vi "MultiStationGasMeter_Rev3.vi"() -> ()   [LabVIEW 2014]
uses:
  <vilib>/DAQmx/read.llb/DAQmx Read (Analog 1D DBL NChan 1Samp).vi
  <vilib>/DAQmx/miscellaneous.llb/DAQmx Fill In Error Info.vi
panel:
  in  "Rate Threshold (V)":dbl=0.02
  in  "HeatingValueLP 3":dbl=990.0 min=900.0 max=2600.0 step=1.0
  in  "HeatingValueNG 3":dbl=990.0 min=900.0 max=1200.0 step=1.0
  in  "Start ANSI 3":bool
  out "ANSI Average (BTU/hr) 3":dbl format="%#_5g"
  out "30 Second Average (BTU/hr) 3":dbl format="%#_5g"
  out "15 Second Average (BTU/hr) 3":dbl format="%#_5g"
  out "Signal 3":bool
  out "CF/HR 3":dbl format="%#_2g"
  out "HV 3":dbl
  out "Meter ID 3":dbl
  out "Gas 3":string
  out "DisplayChart 3":cluster{"Flow Rate":dbl}(graph)
  out "Flow Rate 3":dbl format="%#_5g"
  in  "HeatingValueLP 2":dbl=990.0 min=900.0 max=2600.0 step=1.0
  in  "Start ANSI 2":bool
  out "ANSI Average (BTU/hr) 2":dbl format="%#_5g"
  out "30 Second Average (BTU/hr) 2":dbl format="%#_5g"
  out "15 Second Average (BTU/hr) 2":dbl format="%#_5g"
  out "Signal 2":bool
  out "CF/HR 2":dbl format="%#_2g"
  out "HV 2":dbl
  in  "HeatingValueNG 2":dbl=990.0 min=900.0 max=1200.0 step=1.0
  out "Meter ID 2":dbl
  out "Gas 2":string
  out "DisplayChart 2":cluster{"Flow Rate":dbl}(graph)
  out "Flow Rate 2":dbl format="%#_5g"
  out "ANSI Placeholder 3":dbl
  out "Start Time ANSI 3":dbl
  out "ANSI Placeholder 2":dbl
  out "Start Time ANSI 2":dbl
  out "Meter 6 Present":bool
  out "Meter 5 Present":bool
  out "Meter 4 Present":bool
  out "Meter 3 Present":bool
  out "Meter 2 Present":bool
  out "Meter 1 Present":bool
  out "Meter Type 6":string
  out "Meter Type 2":string
  out "Meter Type 4":string
  out "Meter Type 5":string
  out "Meter Type 3":string
  out "Meter Type 1":string
  out "Meter 6 Size":dbl
  out "Meter 5 Size":dbl
  out "Meter 4 Size":dbl
  out "Meter 3 Size":dbl
  out "Meter 2 Size":dbl
  out "Meter 1 Size":dbl
  out "ANSI Placeholder":dbl
  out "Start Time ANSI":dbl
  in  "Start ANSI":bool
  out "ANSI Average (BTU/hr)":dbl format="%#_5g"
  out "30 Second Average (BTU/hr)":dbl format="%#_5g"
  out "15 Second Average (BTU/hr)":dbl format="%#_5g"
  out "Reference6":dbl
  out "Reference5":dbl
  out "Reference4":dbl
  out "Reference3":dbl
  out "Reference2":dbl
  out "Reference1":dbl
  out "Time":dbl
  out "Num Record":dbl
  in  "HeatingValueLP":dbl=2450.0 min=2400.0 max=2600.0 step=1.0
  out "Output 6":dbl min=0.0 max=5.0 step=0.01
  out "Output 5":dbl min=0.0 max=5.0 step=0.01
  out "Output 4":dbl min=0.0 max=5.0 step=0.01
  out "Output 3":dbl min=0.0 max=5.0 step=0.01
  out "Output 2":dbl min=0.0 max=5.0 step=0.01
  out "Output 1":dbl min=0.0 max=5.0 step=0.01
  out "Signal":bool
  in  "Record":bool
  out "File Path":path
  out "CF/HR":dbl format="%#_2g"
  out "HV":dbl
  in  "HeatingValueNG":dbl=990.0 min=900.0 max=1200.0 step=1.0
  out "Meter ID":dbl
  out "Gas":string
  out "DisplayChart":cluster{"Flow Rate":dbl}(graph)
  out "Flow Rate":dbl format="%#_5g"
  # "STATION 1"
  # "STATION 2"
  # "STATION 3"
  # "Heating Value"
  # "Heating Value"
  # "Heating Value"
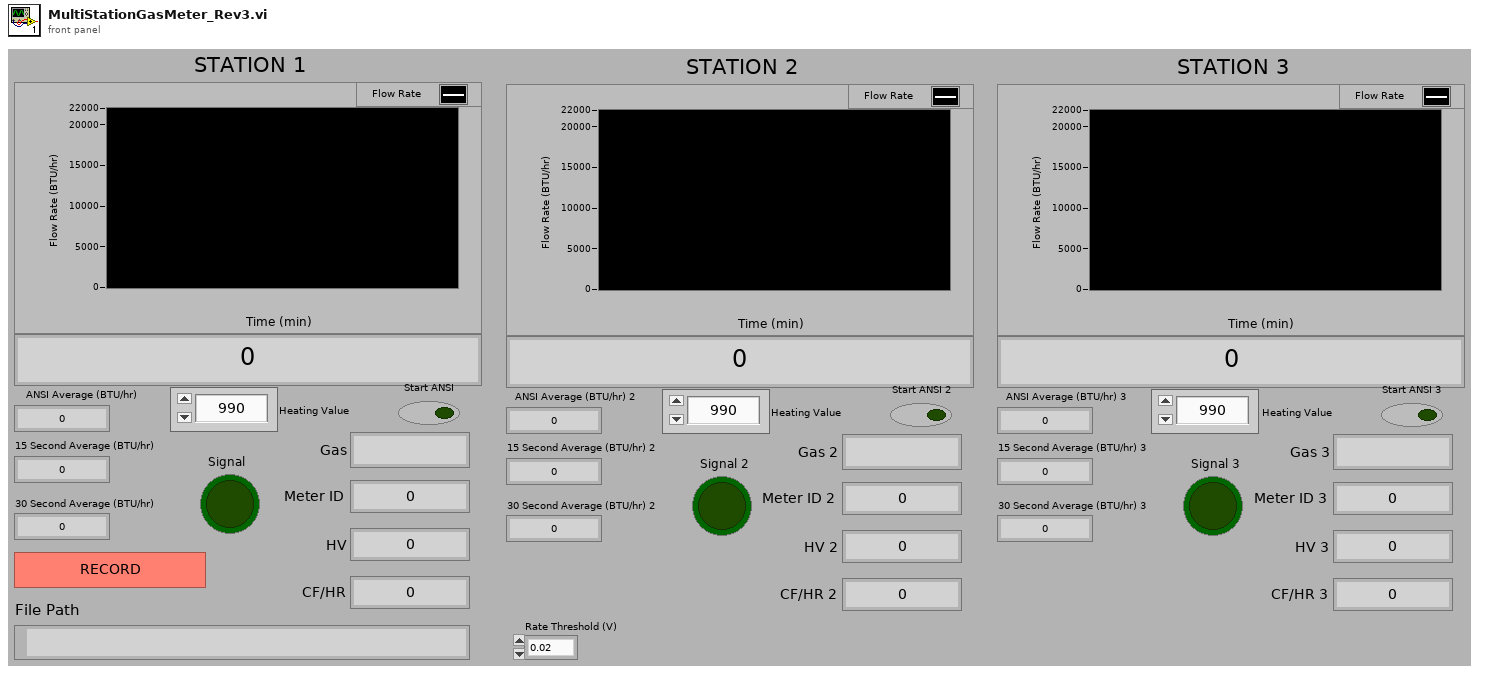
[diagram p1: front panel]
types:
  T1 = enum16{"open", "replace", "create", "open or create", "replace or create", "replace or create with confirmation"}
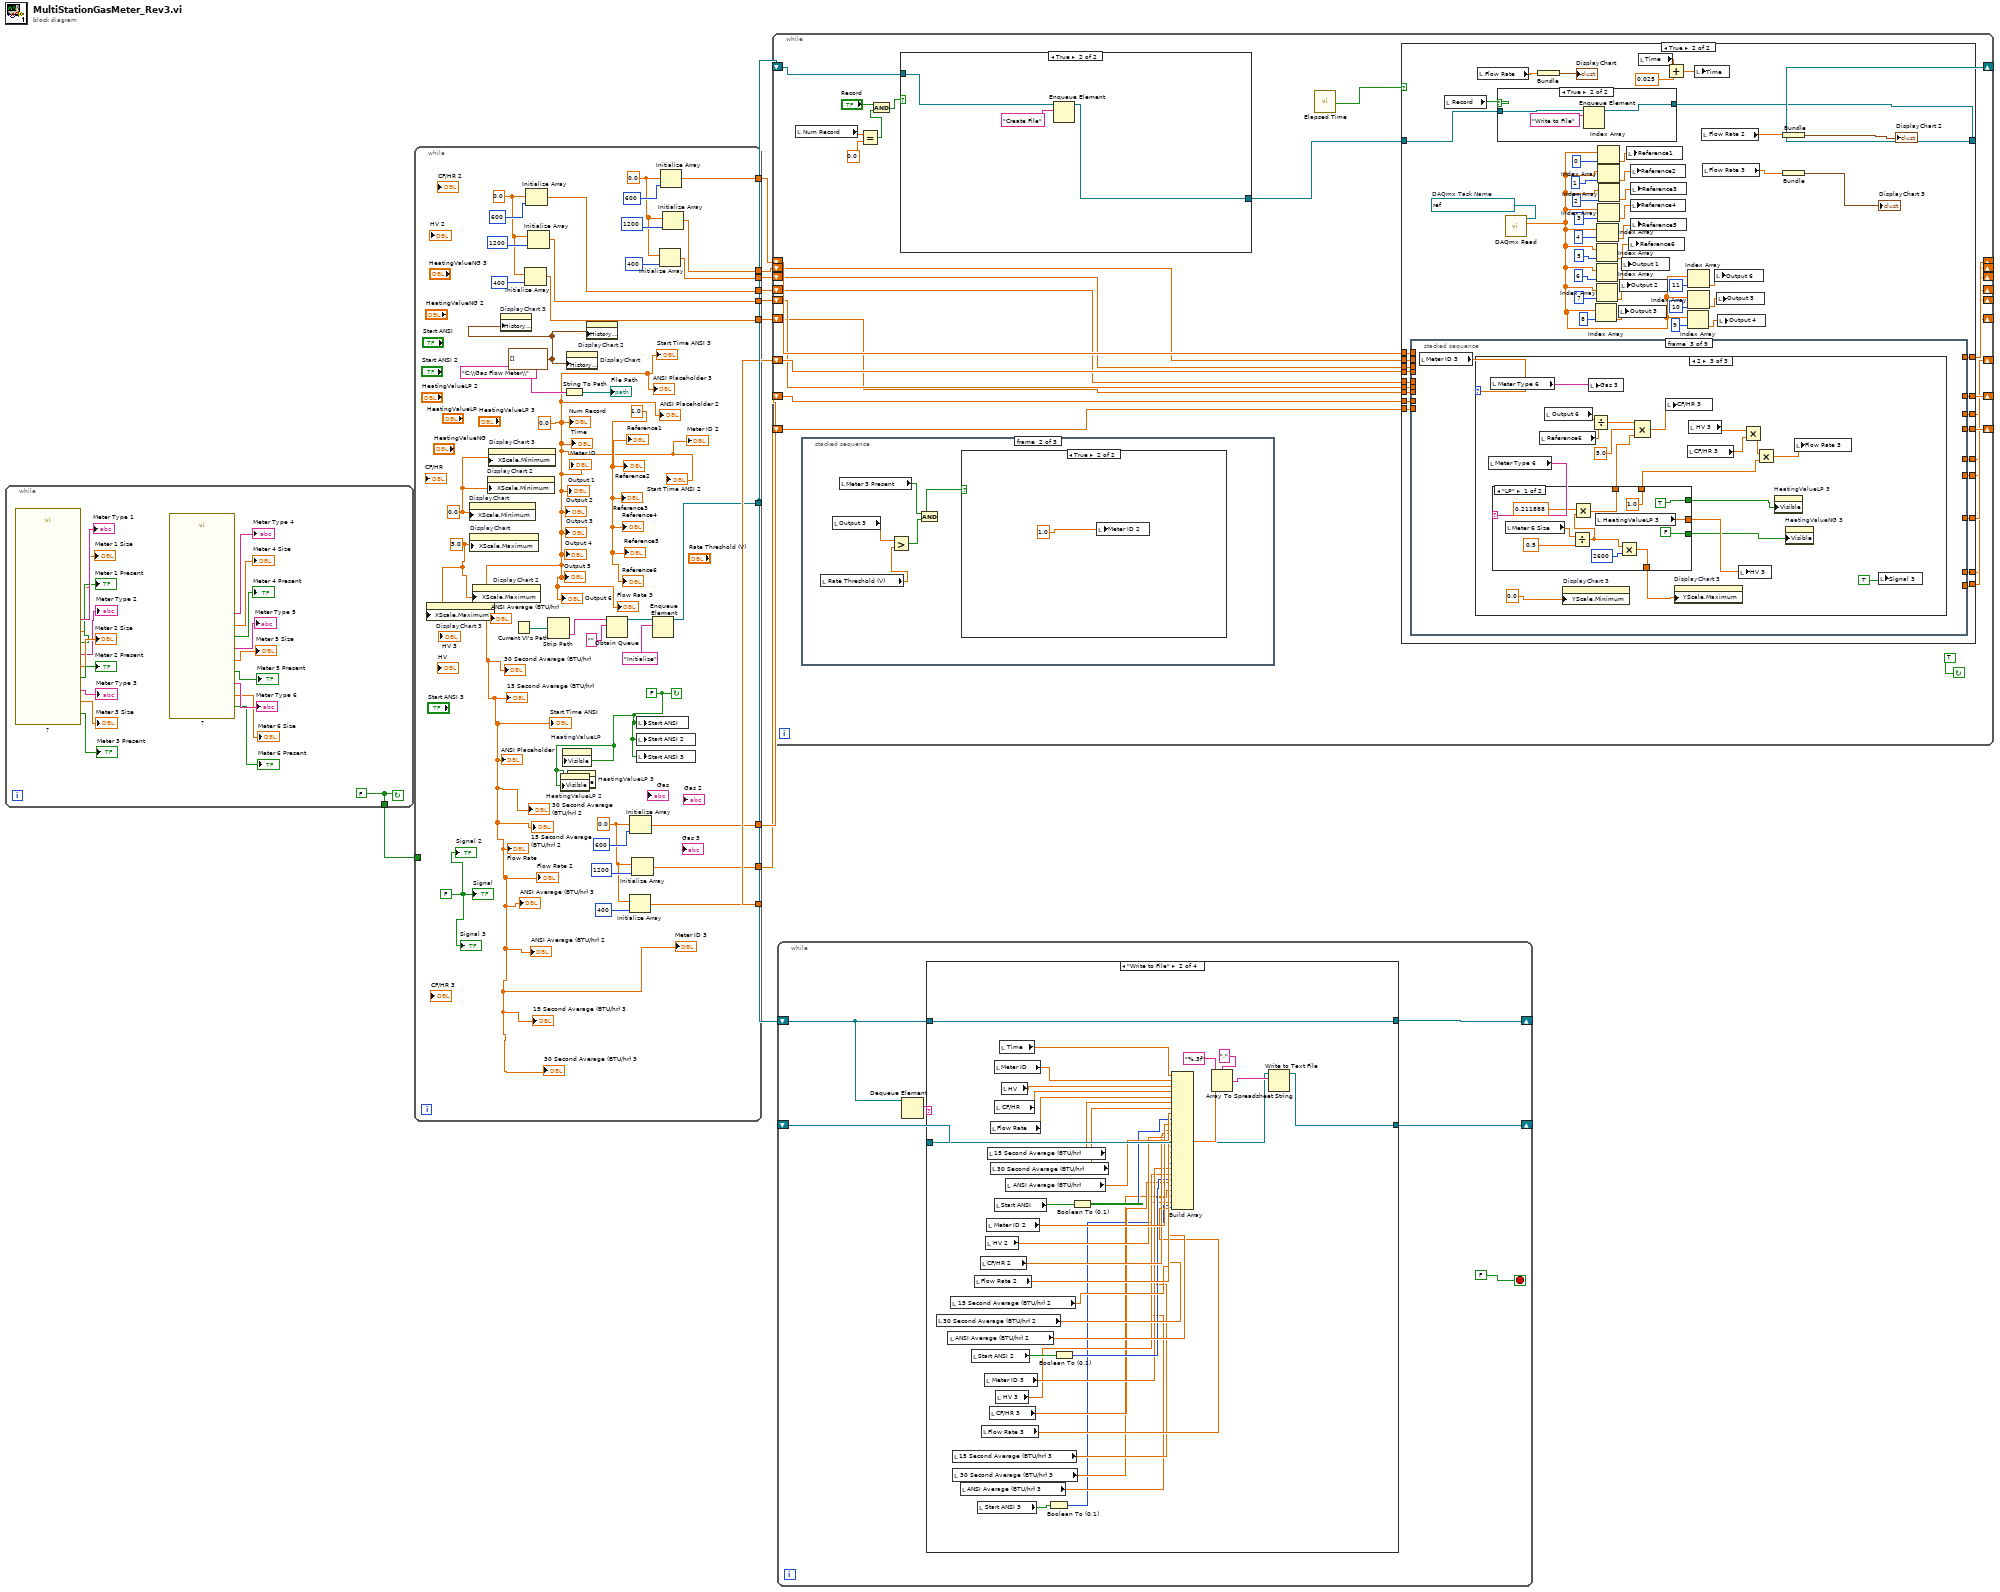
[diagram p0: block diagram]
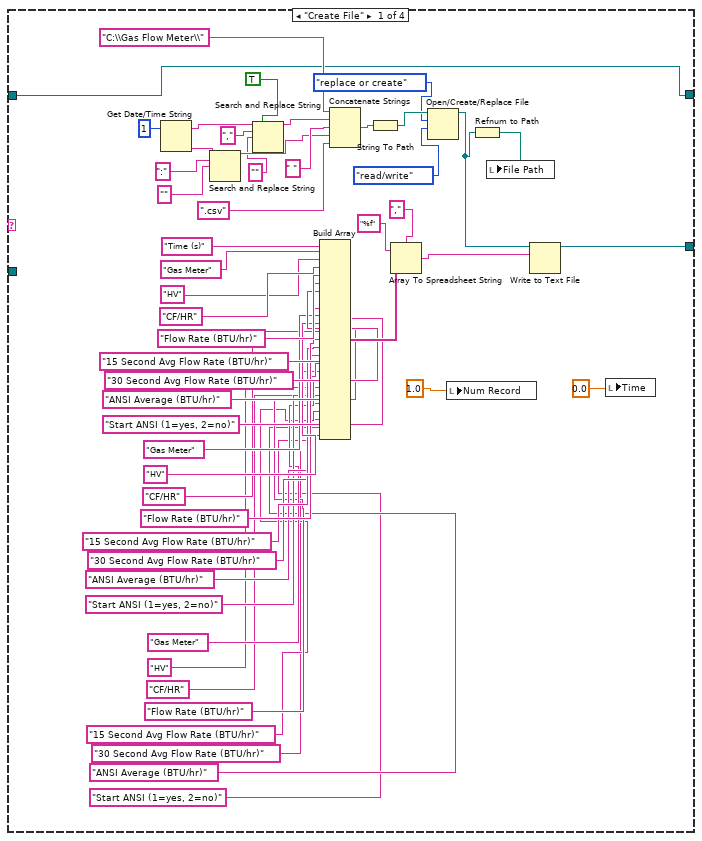
[diagram p2: hidden frame]
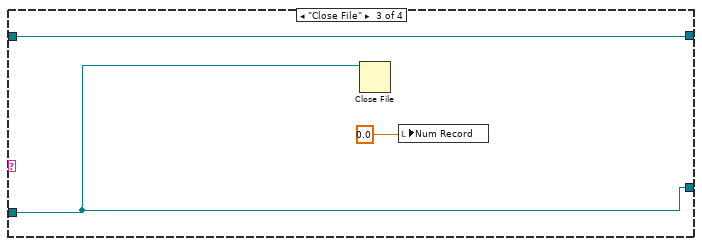
[diagram p3: hidden frame]
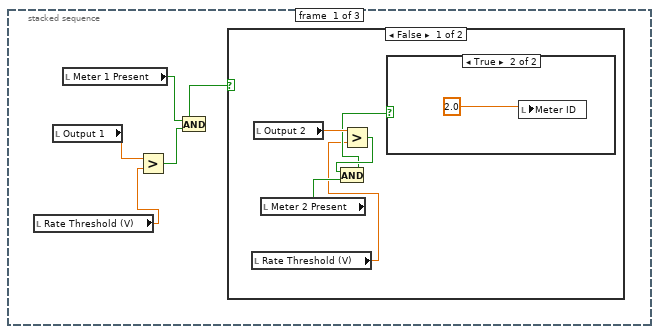
[diagram p5: hidden frame]
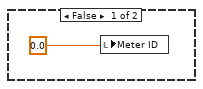
[diagram p6: hidden frame]
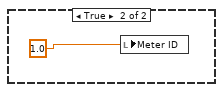
[diagram p7: hidden frame]
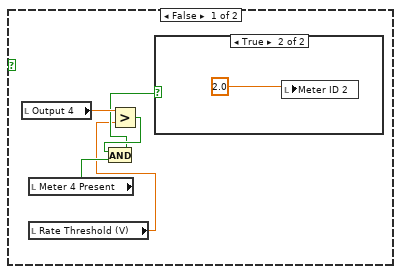
[diagram p8: hidden frame]
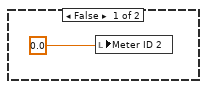
[diagram p9: hidden frame]
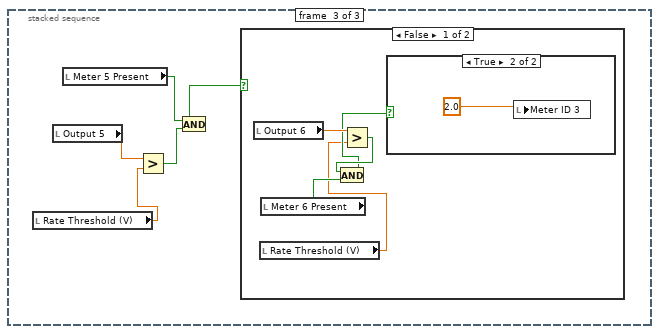
[diagram p10: hidden frame]
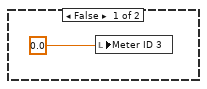
[diagram p11: hidden frame]
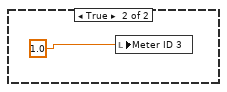
[diagram p12: hidden frame]
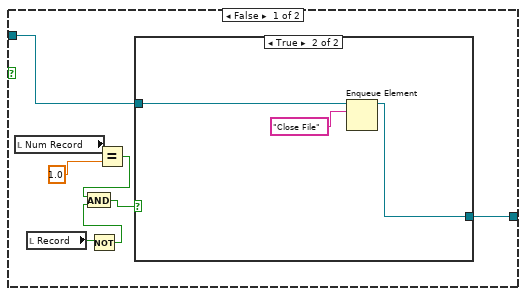
[diagram p13: hidden frame]
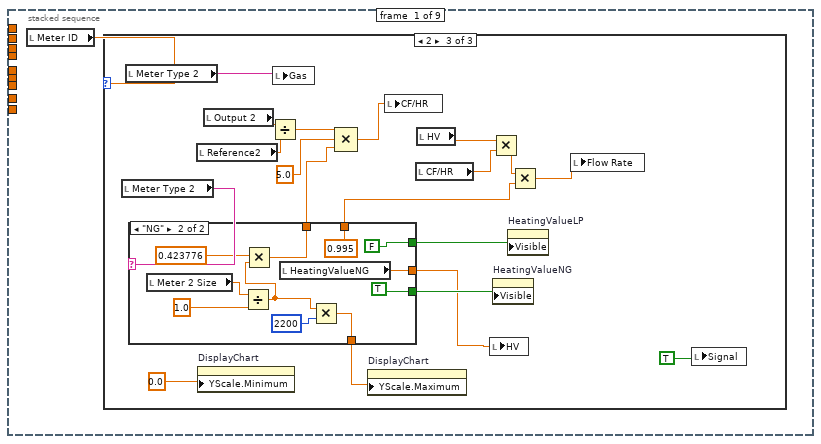
[diagram p16: hidden frame]
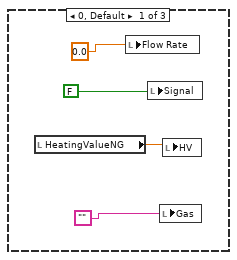
[diagram p17: hidden frame]
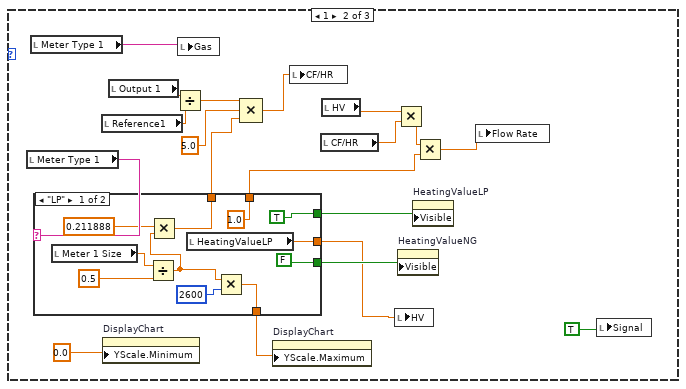
[diagram p18: hidden frame]
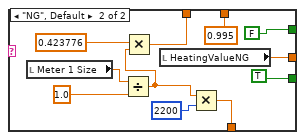
[diagram p19: hidden frame]
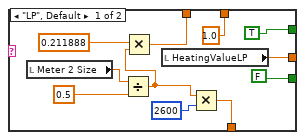
[diagram p20: hidden frame]
diagram:
  n1 = while {
    tunnel: [w29] -> w7
    stop <- w29 continue-if-true
    w29 = FALSE
    n2 = call "?"() -> ("Meter 3 Present?"=→"Meter 3 Present":bool, "Meter Size 3 (SLPM)"=→"Meter 3 Size":dbl, "Meter Type 3 (LP/NG)"=→"Meter Type 3":string, "Meter 2 Present?"=→"Meter 2 Present":bool, "Meter Size 2 (SLPM)"=→"Meter 2 Size":dbl, "Meter Type 2 (LP/NG)"=→"Meter Type 2":string, "Meter 1 Present?"=→"Meter 1 Present":bool, "Meter Size 1 (SLPM)"=→"Meter 1 Size":dbl, "Meter Type 1 (LP/NG)"=→"Meter Type 1":string)  [unwired: 9 in, 2 out]
    n3 = call "?"() -> ("Meter 6 Present?"=→"Meter 6 Present":bool, "Meter Size 6 (SLPM)"=→"Meter 6 Size":dbl, "Meter Type 6 (LP/NG)"=→"Meter Type 6":string, "Meter 5 Present?"=→"Meter 5 Present":bool, "Meter Size 5 (SLPM)"=→"Meter 5 Size":dbl, "Meter Type 5 (LP/NG)"=→"Meter Type 5":string, "Meter 4 Present?"=→"Meter 4 Present":bool, "Meter Size 4 (SLPM)"=→"Meter 4 Size":dbl, "Meter Type 4 (LP/NG)"=→"Meter Type 4":string)  [unwired: 9 in, 2 out]
  }
  n4 = while {
    tunnel: [w60] -> w11
    tunnel: [w56] -> w10
    tunnel: [w55] -> w9
    tunnel: [w52] -> w8
    tunnel: w7 -> [_]
    tunnel: [w47] -> w6
    tunnel: [w46] -> w5
    tunnel: [w45] -> w4
    tunnel: [w40] -> w3
    tunnel: [w39] -> w2
    tunnel: [w38] -> w1
    stop <- w36 continue-if-true
    w42 = 0.0
    w49 = 0.0
    w35 = FALSE
    w54 = 0.0
    w31 = 5.0
    w32 = 0.0
    w59 = 1.0
    w34 = 0.0
    w33 = cluster{"[0]":dbl}[] []
    w36 = FALSE
    n5 = property on="DisplayChart 3" class="WFChart (strict)"("XScale.Maximum"=w31) -> ()  [unwired: 2 in, 2 out]
    n6 = property on="DisplayChart" class="WFChart (strict)"("XScale.Minimum"=w32) -> ()  [unwired: 2 in, 2 out]
    n7 = property on="DisplayChart" class="WFChart (strict)"("XScale.Maximum"=w31) -> ()  [unwired: 2 in, 2 out]
    n8 = property on="DisplayChart 2" class="WFChart (strict)"("XScale.Maximum"=w31) -> ()  [unwired: 2 in, 2 out]
    n9 = property on="DisplayChart 2" class="WFChart (strict)"("XScale.Minimum"=w32) -> ()  [unwired: 2 in, 2 out]
    n10 = property on="DisplayChart 3" class="WFChart (strict)"("XScale.Minimum"=w32) -> ()  [unwired: 2 in, 2 out]
    n11 = property on="DisplayChart 3" class="WFChart (strict)"("History Data"=w33) -> ()  [unwired: 2 in, 2 out]
    n12 = Current VI's Path() -> (path=w65:path)
    n13 = Initialize Array(w42, 400) -> (w38:dbl[])
    n14 = Initialize Array(w42, 600) -> (w40:dbl[])
    n15 = Initialize Array(w42, 1200) -> (w39:dbl[])
    n16 = Strip Path(path=w65) -> (name=w63:string)  [unwired: 1 out]
    n17 = property on="HeatingValueLP 2" class="DigNum (strict)"("Visible"=w36) -> ()  [unwired: 2 in, 2 out]
    n18 = property on="HeatingValueLP" class="DigNum (strict)"("Visible"=w36) -> ()  [unwired: 2 in, 2 out]
    n19 = String To Path(string="C:\\Gas Flow Meter\\") -> (path=→"File Path":path)
    n20 = property on="DisplayChart" class="WFChart (strict)"("History Data"=w33) -> ()  [unwired: 2 in, 2 out]
    n21 = property on="HeatingValueLP 3" class="DigNum (strict)"("Visible"=w36) -> ()  [unwired: 2 in, 2 out]
    n22 = property on="DisplayChart 2" class="WFChart (strict)"("History Data"=w33) -> ()  [unwired: 2 in, 2 out]
    n23 = Obtain Queue(name (unnamed)=w63, element data type="") -> (queue out=w61:refnum<queue>)  [unwired: 3 in, 2 out]
    n24 = Initialize Array(w54, 400) -> (w52:dbl[])
    n25 = Initialize Array(w54, 600) -> (w56:dbl[])
    n26 = Initialize Array(w54, 1200) -> (w55:dbl[])
    n27 = local write "Start ANSI"(w36) -> ()
    n28 = local write "Start ANSI 2"(w36) -> ()
    n29 = local write "Start ANSI 3"(w36) -> ()
    n30 = Enqueue Element(queue=w61, element="Initialize") -> (queue out=w60:refnum<queue>)  [unwired: 2 in, 2 out]
    n31 = Initialize Array(w49, 400) -> (w45:dbl[])
    n32 = Initialize Array(w49, 600) -> (w47:dbl[])
    n33 = Initialize Array(w49, 1200) -> (w46:dbl[])
    "Num Record" <- w34
    "Time" <- w34
    "Meter ID" <- w34
    "Output 1" <- w34
    "Output 2" <- w34
    "Output 3" <- w34
    "Output 4" <- w34
    "Output 5" <- w34
    "Output 6" <- w34
    "Reference1" <- w59
    "Reference2" <- w59
    "Reference3" <- w59
    "Reference4" <- w59
    "Reference5" <- w59
    "Reference6" <- w59
    "30 Second Average (BTU/hr)" <- w34
    "15 Second Average (BTU/hr)" <- w34
    "ANSI Average (BTU/hr)" <- w34
    "Start Time ANSI" <- w34
    "ANSI Placeholder" <- w34
    "Flow Rate" <- w34
    "Signal" <- w35
    "Start Time ANSI 3" <- w34
    "ANSI Placeholder 3" <- w34
    "ANSI Placeholder 2" <- w34
    "Start Time ANSI 2" <- w34
    "Signal 2" <- w35
    "Flow Rate 2" <- w34
    "ANSI Average (BTU/hr) 2" <- w34
    "Meter ID 2" <- w34
    "30 Second Average (BTU/hr) 2" <- w34
    "15 Second Average (BTU/hr) 2" <- w34
    "Signal 3" <- w35
    "Flow Rate 3" <- w34
    "Meter ID 3" <- w34
    "ANSI Average (BTU/hr) 3" <- w34
    "15 Second Average (BTU/hr) 3" <- w34
    "30 Second Average (BTU/hr) 3" <- w34
  }
  n34 = while {
    shift-right: [w92] -> _
    shift-left: w11 -> [w85]
    shift-right: [w91] -> _
    shift-left: w10 -> [w89]
    shift-right: [w90] -> _
    shift-left: w9 -> [w88]
    shift-right: [w87] -> _
    shift-left: w8 -> [w86]
    shift-right: [w77] -> _
    shift-left: w6 -> [w78]
    shift-right: [w75] -> _
    shift-left: w5 -> [w76]
    shift-right: [w73] -> _
    shift-left: w4 -> [w74]
    shift-right: [w71] -> _
    shift-left: w3 -> [w72]
    shift-right: [w69] -> _
    shift-left: w2 -> [w70]
    shift-right: [w67] -> _
    shift-left: w1 -> [w68]
    stop <- TRUE continue-if-true
    n35 = local read "Num Record"() -> (w81:dbl)
    n36 = stacked-sequence {
      frame #0 {
        n37 = local read "Rate Threshold (V)"() -> (w95:dbl)
        n38 = local read "Output 1"() -> (w99:dbl)
        n39 = local read "Meter 1 Present"() -> (w97:bool)
        n40 = Greater?(x=w99, y=w95) -> (0:w98:bool)
        n41 = And(x=w97, y=w98) -> (x .and. y?=w96:bool)
        n42 = case shown="False" w96 {
          frame False {
            n43 = local read "Rate Threshold (V)"() -> (w100:dbl)
            n44 = local read "Output 2"() -> (w104:dbl)
            n45 = local read "Meter 2 Present"() -> (w103:bool)
            n46 = Greater?(x=w104, y=w100) -> (0:w102:bool)
            n47 = And(x=w102, y=w103) -> (x .and. y?=w101:bool)
            n48 = case shown="True" w101 {
              frame False {
                n49 = local write "Meter ID"(0.0) -> ()
              }
              frame True {
                n50 = local write "Meter ID"(2.0) -> ()
              }
            }
          }
          frame True {
            n51 = local write "Meter ID"(1.0) -> ()
          }
        }
      }
      frame #1 {
        n52 = local read "Rate Threshold (V)"() -> (w108:dbl)
        n53 = local read "Output 3"() -> (w112:dbl)
        n54 = local read "Meter 3 Present"() -> (w110:bool)
        n55 = Greater?(x=w112, y=w108) -> (0:w111:bool)
        n56 = And(x=w110, y=w111) -> (x .and. y?=w109:bool)
        n57 = case shown="True" w109 {
          frame False {
            n58 = local read "Output 4"() -> (w117:dbl)
            n59 = local read "Meter 4 Present"() -> (w116:bool)
            n60 = local read "Rate Threshold (V)"() -> (w113:dbl)
            n61 = Greater?(x=w117, y=w113) -> (0:w115:bool)
            n62 = And(x=w115, y=w116) -> (x .and. y?=w114:bool)
            n63 = case shown="True" w114 {
              frame False {
                n64 = local write "Meter ID 2"(0.0) -> ()
              }
              frame True {
                n65 = local write "Meter ID 2"(2.0) -> ()
              }
            }
          }
          frame True {
            n66 = local write "Meter ID 2"(1.0) -> ()
          }
        }
      }
      frame #2 {
        n67 = local read "Rate Threshold (V)"() -> (w121:dbl)
        n68 = local read "Output 5"() -> (w125:dbl)
        n69 = local read "Meter 5 Present"() -> (w123:bool)
        n70 = Greater?(x=w125, y=w121) -> (0:w124:bool)
        n71 = And(x=w123, y=w124) -> (x .and. y?=w122:bool)
        n72 = case shown="False" w122 {
          frame False {
            n73 = local read "Output 6"() -> (w130:dbl)
            n74 = local read "Rate Threshold (V)"() -> (w126:dbl)
            n75 = local read "Meter 6 Present"() -> (w129:bool)
            n76 = Greater?(x=w130, y=w126) -> (0:w128:bool)
            n77 = And(x=w128, y=w129) -> (x .and. y?=w127:bool)
            n78 = case shown="True" w127 {
              frame False {
                n79 = local write "Meter ID 3"(0.0) -> ()
              }
              frame True {
                n80 = local write "Meter ID 3"(2.0) -> ()
              }
            }
          }
          frame True {
            n81 = local write "Meter ID 3"(1.0) -> ()
          }
        }
      }
    }
    n82 = Equal?(x=w81, y=0.0) -> (x = y?=w80:bool)
    n83 = And(x="Record", y=w80) -> (x .and. y?=w79:bool)
    n84 = case shown="True" w79 {
      tunnel: w85 -> [w139 w147]
      tunnel: [w138 w146] -> w84
      frame False {
        n85 = local read "Num Record"() -> (w141:dbl)
        n86 = local read "Record"() -> (w135:bool)
        n87 = Not(x=w135) -> (.not. x?=w134:bool)
        n88 = Equal?(x=w141, y=1.0) -> (x = y?=w137:bool)
        n89 = And(x=w137, y=w134) -> (x .and. y?=w136:bool)
        n90 = case shown="True" w136 {
          tunnel: w139 -> [w142 w144]
          tunnel: [w142 w143] -> w138
          frame False {
          }
          frame True {
            n91 = Enqueue Element(queue=w144, element="Close File") -> (queue out=w143:refnum<queue>)  [unwired: 2 in, 2 out]
          }
        }
      }
      frame True {
        n92 = Enqueue Element(queue=w147, element="Create File") -> (queue out=w146:refnum<queue>)  [unwired: 2 in, 2 out]
      }
    }
    n93 = call "Elapsed Time"() -> ("Time has Elapsed"=w93:bool)  [unwired: 12 in, 7 out]
    n94 = case shown="True" w93 {
      tunnel: w84 -> [w158 w208]
      tunnel: [w158 w207] -> w92
      tunnel: w89 -> [w157 w180]
      tunnel: w88 -> [w156 w179]
      tunnel: [w157 w178] -> w91
      tunnel: [w156 w177] -> w90
      tunnel: w86 -> [w155 w176]
      tunnel: [w155 w175] -> w87
      tunnel: w78 -> [w152 w174]
      tunnel: [w152 w173] -> w77
      tunnel: w76 -> [w153 w172]
      tunnel: [w153 w171] -> w75
      tunnel: w74 -> [w154 w170]
      tunnel: [w154 w169] -> w73
      tunnel: w72 -> [w151 w168]
      tunnel: [w151 w167] -> w71
      tunnel: w70 -> [w150 w166]
      tunnel: [w150 w165] -> w69
      tunnel: w68 -> [w149 w164]
      tunnel: [w149 w163] -> w67
      frame False {
      }
      frame True {
        w206 = refnum<k21> "ReadFlowMeterIn"  # DAQmx Task Name
        n95 = stacked-sequence {
          tunnel: w180 -> [_ _ _ w500 _ _ _ _ _]
          tunnel: w179 -> [_ _ _ w499 _ _ _ _ _]
          tunnel: [_ _ _ w494 _ _ _ _ _] -> w178
          tunnel: [_ _ _ w490 _ _ _ _ _] -> w177
          tunnel: w176 -> [_ _ _ w484 _ _ _ _ _]
          tunnel: [_ _ _ w481 _ _ _ _ _] -> w175
          tunnel: w174 -> [_ _ _ _ w523 _ _ _ _]
          tunnel: [_ _ _ _ w510 _ _ _ _] -> w173
          tunnel: w172 -> [_ _ _ _ w517 _ _ _ _]
          tunnel: [_ _ _ _ w509 _ _ _ _] -> w171
          tunnel: w170 -> [_ _ _ _ w515 _ _ _ _]
          tunnel: [_ _ _ _ w508 _ _ _ _] -> w169
          tunnel: w168 -> [_ _ _ _ _ w544 _ _ _]
          tunnel: [_ _ _ _ _ w542 _ _ _] -> w167
          tunnel: w166 -> [_ _ _ _ _ w541 _ _ _]
          tunnel: [_ _ _ _ _ w539 _ _ _] -> w165
          tunnel: w164 -> [_ _ _ _ _ w538 _ _ _]
          tunnel: [_ _ _ _ _ w536 _ _ _] -> w163
          frame #0 {
            n96 = local read "Meter ID"() -> (w215:dbl)
            n97 = case shown="2" w215 {
              frame 0, Default {
                n98 = local read "HeatingValueNG"() -> (w219:dbl)
                n99 = local write "Flow Rate"(0.0) -> ()
                n100 = local write "Signal"(FALSE) -> ()
                n101 = local write "Gas"("") -> ()
                n102 = local write "HV"(w219) -> ()
              }
              frame 1 {
                n103 = local read "Meter Type 1"() -> (w228:string)
                n104 = local read "Meter Type 1"() -> (w222:string)
                n105 = case shown="\"LP\"" w228 {
                  tunnel: [w246 w257] -> w227
                  tunnel: [TRUE FALSE] -> w226
                  tunnel: [FALSE TRUE] -> w225
                  tunnel: [1.0 0.995] -> w224
                  tunnel: [w240 w251] -> w223
                  tunnel: [w239 w250] -> w221
                  frame "LP" {
                    n106 = local read "Meter 1 Size"() -> (w248:dbl)
                    n107 = Divide(x=w248, y=0.5) -> (x/y=w241:dbl)
                    n108 = Multiply(x=0.211888, y=w241) -> (x*y=w246:dbl)
                    n109 = local read "HeatingValueLP"() -> (w239:dbl)
                    n110 = Multiply(x=w241, y=2600) -> (x*y=w240:dbl)
                  }
                  frame "NG", Default {
                    n111 = local read "Meter 1 Size"() -> (w259:dbl)
                    n112 = Divide(x=w259, y=1.0) -> (x/y=w252:dbl)
                    n113 = Multiply(x=0.423776, y=w252) -> (x*y=w257:dbl)
                    n114 = local read "HeatingValueNG"() -> (w250:dbl)
                    n115 = Multiply(x=w252, y=2200) -> (x*y=w251:dbl)
                  }
                }
                n116 = local read "Reference1"() -> (w232:dbl)
                n117 = property on="DisplayChart" class="WFChart (strict)"("YScale.Minimum"=0.0) -> ()  [unwired: 2 in, 2 out]
                n118 = local read "Output 1"() -> (w233:dbl)
                n119 = Divide(x=w233, y=w232) -> (x/y=w230:dbl)
                n120 = local write "Gas"(w222) -> ()
                n121 = Compound Arithmetic op=MULTIPLY(w230, 5.0, w227) -> (w220:dbl)
                n122 = property on="DisplayChart" class="WFChart (strict)"("YScale.Maximum"=w223) -> ()  [unwired: 2 in, 2 out]
                n123 = local write "CF/HR"(w220) -> ()
                n124 = local read "CF/HR"() -> (w235:dbl)
                n125 = local read "HV"() -> (w234:dbl)
                n126 = local write "HV"(w221) -> ()
                n127 = Multiply(x=w234, y=w235) -> (x*y=w236:dbl)
                n128 = property on="HeatingValueNG" class="DigNum (strict)"("Visible"=w225) -> ()  [unwired: 2 in, 2 out]
                n129 = property on="HeatingValueLP" class="DigNum (strict)"("Visible"=w226) -> ()  [unwired: 2 in, 2 out]
                n130 = Multiply(x=w236, y=w224) -> (x*y=w237:dbl)
                n131 = local write "Flow Rate"(w237) -> ()
                n132 = local write "Signal"(TRUE) -> ()
              }
              frame 2 {
                n133 = local read "Meter Type 2"() -> (w269:string)
                n134 = local read "Meter Type 2"() -> (w263:string)
                n135 = case shown="\"NG\"" w269 {
                  tunnel: [w287 w298] -> w268
                  tunnel: [TRUE FALSE] -> w267
                  tunnel: [FALSE TRUE] -> w266
                  tunnel: [1.0 0.995] -> w265
                  tunnel: [w281 w292] -> w264
                  tunnel: [w280 w291] -> w262
                  frame "LP", Default {
                    n136 = local read "Meter 2 Size"() -> (w289:dbl)
                    n137 = Divide(x=w289, y=0.5) -> (x/y=w282:dbl)
                    n138 = Multiply(x=0.211888, y=w282) -> (x*y=w287:dbl)
                    n139 = local read "HeatingValueLP"() -> (w280:dbl)
                    n140 = Multiply(x=w282, y=2600) -> (x*y=w281:dbl)
                  }
                  frame "NG" {
                    n141 = local read "Meter 2 Size"() -> (w300:dbl)
                    n142 = Divide(x=w300, y=1.0) -> (x/y=w293:dbl)
                    n143 = Multiply(x=0.423776, y=w293) -> (x*y=w298:dbl)
                    n144 = local read "HeatingValueNG"() -> (w291:dbl)
                    n145 = Multiply(x=w293, y=2200) -> (x*y=w292:dbl)
                  }
                }
                n146 = local read "Reference2"() -> (w273:dbl)
                n147 = property on="DisplayChart" class="WFChart (strict)"("YScale.Minimum"=0.0) -> ()  [unwired: 2 in, 2 out]
                n148 = local read "Output 2"() -> (w274:dbl)
                n149 = Divide(x=w274, y=w273) -> (x/y=w271:dbl)
                n150 = local write "Gas"(w263) -> ()
                n151 = Compound Arithmetic op=MULTIPLY(w271, 5.0, w268) -> (w261:dbl)
                n152 = property on="DisplayChart" class="WFChart (strict)"("YScale.Maximum"=w264) -> ()  [unwired: 2 in, 2 out]
                n153 = local write "CF/HR"(w261) -> ()
                n154 = local read "CF/HR"() -> (w276:dbl)
                n155 = local read "HV"() -> (w275:dbl)
                n156 = local write "HV"(w262) -> ()
                n157 = Multiply(x=w275, y=w276) -> (x*y=w277:dbl)
                n158 = property on="HeatingValueNG" class="DigNum (strict)"("Visible"=w266) -> ()  [unwired: 2 in, 2 out]
                n159 = property on="HeatingValueLP" class="DigNum (strict)"("Visible"=w267) -> ()  [unwired: 2 in, 2 out]
                n160 = Multiply(x=w277, y=w265) -> (x*y=w278:dbl)
                n161 = local write "Flow Rate"(w278) -> ()
                n162 = local write "Signal"(TRUE) -> ()
              }
            }
          }
          frame #1 {
            n163 = local read "Meter ID 2"() -> (w302:dbl)
            n164 = case shown="0, Default" w302 {
              frame 0, Default {
                n165 = local read "HeatingValueNG 2"() -> (w306:dbl)
                n166 = local write "Flow Rate 2"(0.0) -> ()
                n167 = local write "Signal 2"(FALSE) -> ()
                n168 = local write "Gas 2"("") -> ()
                n169 = local write "HV 2"(w306) -> ()
              }
              frame 1 {
                n170 = local read "Meter Type 3"() -> (w316:string)
                n171 = local read "Meter Type 3"() -> (w313:string)
                n172 = case shown="\"LP\"" w316 {
                  tunnel: [w333 w344] -> w315
                  tunnel: [TRUE FALSE] -> w309
                  tunnel: [FALSE TRUE] -> w310
                  tunnel: [1.0 0.995] -> w314
                  tunnel: [w327 w338] -> w307
                  tunnel: [w326 w337] -> w312
                  frame "LP" {
                    n173 = local read "Meter 3 Size"() -> (w335:dbl)
                    n174 = Divide(x=w335, y=0.5) -> (x/y=w328:dbl)
                    n175 = Multiply(x=0.211888, y=w328) -> (x*y=w333:dbl)
                    n176 = local read "HeatingValueLP 2"() -> (w326:dbl)
                    n177 = Multiply(x=w328, y=2600) -> (x*y=w327:dbl)
                  }
                  frame "NG", Default {
                    n178 = local read "Meter 3 Size"() -> (w346:dbl)
                    n179 = Divide(x=w346, y=1.0) -> (x/y=w339:dbl)
                    n180 = Multiply(x=0.423776, y=w339) -> (x*y=w344:dbl)
                    n181 = local read "HeatingValueNG 2"() -> (w337:dbl)
                    n182 = Multiply(x=w339, y=2200) -> (x*y=w338:dbl)
                  }
                }
                n183 = local read "Reference3"() -> (w319:dbl)
                n184 = local read "Output 3"() -> (w320:dbl)
                n185 = property on="DisplayChart 2" class="WFChart (strict)"("YScale.Minimum"=0.0) -> ()  [unwired: 2 in, 2 out]
                n186 = local write "Gas 2"(w313) -> ()
                n187 = Divide(x=w320, y=w319) -> (x/y=w317:dbl)
                n188 = Compound Arithmetic op=MULTIPLY(w317, 5.0, w315) -> (w311:dbl)
                n189 = local write "CF/HR 2"(w311) -> ()
                n190 = property on="DisplayChart 2" class="WFChart (strict)"("YScale.Maximum"=w307) -> ()  [unwired: 2 in, 2 out]
                n191 = local read "CF/HR 2"() -> (w322:dbl)
                n192 = local read "HV 2"() -> (w321:dbl)
                n193 = local write "HV 2"(w312) -> ()
                n194 = Multiply(x=w321, y=w322) -> (x*y=w323:dbl)
                n195 = Multiply(x=w323, y=w314) -> (x*y=w324:dbl)
                n196 = property on="HeatingValueLP 2" class="DigNum (strict)"("Visible"=w309) -> ()  [unwired: 2 in, 2 out]
                n197 = property on="HeatingValueNG 2" class="DigNum (strict)"("Visible"=w310) -> ()  [unwired: 2 in, 2 out]
                n198 = local write "Flow Rate 2"(w324) -> ()
                n199 = local write "Signal 2"(TRUE) -> ()
              }
              frame 2 {
                n200 = local read "Meter Type 4"() -> (w357:string)
                n201 = local read "Meter Type 4"() -> (w354:string)
                n202 = case shown="\"LP\"" w357 {
                  tunnel: [w374 w385] -> w356
                  tunnel: [TRUE FALSE] -> w350
                  tunnel: [FALSE TRUE] -> w351
                  tunnel: [1.0 0.995] -> w355
                  tunnel: [w368 w379] -> w348
                  tunnel: [w367 w378] -> w353
                  frame "LP" {
                    n203 = local read "Meter 4 Size"() -> (w376:dbl)
                    n204 = Divide(x=w376, y=0.5) -> (x/y=w369:dbl)
                    n205 = Multiply(x=0.211888, y=w369) -> (x*y=w374:dbl)
                    n206 = local read "HeatingValueLP 2"() -> (w367:dbl)
                    n207 = Multiply(x=w369, y=2600) -> (x*y=w368:dbl)
                  }
                  frame "NG", Default {
                    n208 = local read "Meter 3 Size"() -> (w387:dbl)
                    n209 = Divide(x=w387, y=1.0) -> (x/y=w380:dbl)
                    n210 = Multiply(x=0.423776, y=w380) -> (x*y=w385:dbl)
                    n211 = local read "HeatingValueNG 2"() -> (w378:dbl)
                    n212 = Multiply(x=w380, y=2200) -> (x*y=w379:dbl)
                  }
                }
                n213 = local read "Reference4"() -> (w360:dbl)
                n214 = local read "Output 4"() -> (w361:dbl)
                n215 = property on="DisplayChart 2" class="WFChart (strict)"("YScale.Minimum"=0.0) -> ()  [unwired: 2 in, 2 out]
                n216 = local write "Gas 2"(w354) -> ()
                n217 = Divide(x=w361, y=w360) -> (x/y=w358:dbl)
                n218 = Compound Arithmetic op=MULTIPLY(w358, 5.0, w356) -> (w352:dbl)
                n219 = local write "CF/HR 2"(w352) -> ()
                n220 = property on="DisplayChart 2" class="WFChart (strict)"("YScale.Maximum"=w348) -> ()  [unwired: 2 in, 2 out]
                n221 = local read "CF/HR 2"() -> (w363:dbl)
                n222 = local read "HV 2"() -> (w362:dbl)
                n223 = local write "HV 2"(w353) -> ()
                n224 = Multiply(x=w362, y=w363) -> (x*y=w364:dbl)
                n225 = Multiply(x=w364, y=w355) -> (x*y=w365:dbl)
                n226 = property on="HeatingValueLP 2" class="DigNum (strict)"("Visible"=w350) -> ()  [unwired: 2 in, 2 out]
                n227 = property on="HeatingValueNG 2" class="DigNum (strict)"("Visible"=w351) -> ()  [unwired: 2 in, 2 out]
                n228 = local write "Flow Rate 2"(w365) -> ()
                n229 = local write "Signal 2"(TRUE) -> ()
              }
            }
          }
          frame #2 {
            n230 = local read "Meter ID 3"() -> (w389:dbl)
            n231 = case shown="2" w389 {
              frame 0, Default {
                n232 = local read "HeatingValueNG 3"() -> (w393:dbl)
                n233 = local write "Flow Rate 3"(0.0) -> ()
                n234 = local write "Signal 3"(FALSE) -> ()
                n235 = local write "Gas 3"("") -> ()
                n236 = local write "HV 3"(w393) -> ()
              }
              frame 1 {
                n237 = local read "Meter Type 5"() -> (w403:string)
                n238 = local read "Meter Type 5"() -> (w400:string)
                n239 = case shown="\"LP\"" w403 {
                  tunnel: [w420 w431] -> w402
                  tunnel: [TRUE FALSE] -> w396
                  tunnel: [FALSE TRUE] -> w397
                  tunnel: [1.0 0.995] -> w401
                  tunnel: [w414 w425] -> w395
                  tunnel: [w413 w424] -> w399
                  frame "LP" {
                    n240 = local read "Meter 5 Size"() -> (w422:dbl)
                    n241 = Divide(x=w422, y=0.5) -> (x/y=w415:dbl)
                    n242 = Multiply(x=0.211888, y=w415) -> (x*y=w420:dbl)
                    n243 = local read "HeatingValueLP 3"() -> (w413:dbl)
                    n244 = Multiply(x=w415, y=2600) -> (x*y=w414:dbl)
                  }
                  frame "NG", Default {
                    n245 = local read "Meter 5 Size"() -> (w433:dbl)
                    n246 = Divide(x=w433, y=1.0) -> (x/y=w426:dbl)
                    n247 = Multiply(x=0.423776, y=w426) -> (x*y=w431:dbl)
                    n248 = local read "HeatingValueNG 3"() -> (w424:dbl)
                    n249 = Multiply(x=w426, y=2200) -> (x*y=w425:dbl)
                  }
                }
                n250 = local read "Reference5"() -> (w406:dbl)
                n251 = local read "Output 5"() -> (w407:dbl)
                n252 = property on="DisplayChart 3" class="WFChart (strict)"("YScale.Minimum"=0.0) -> ()  [unwired: 2 in, 2 out]
                n253 = local write "Gas 3"(w400) -> ()
                n254 = Divide(x=w407, y=w406) -> (x/y=w404:dbl)
                n255 = Compound Arithmetic op=MULTIPLY(w404, 5.0, w402) -> (w398:dbl)
                n256 = local write "CF/HR 3"(w398) -> ()
                n257 = property on="DisplayChart 3" class="WFChart (strict)"("YScale.Maximum"=w395) -> ()  [unwired: 2 in, 2 out]
                n258 = local read "CF/HR 3"() -> (w409:dbl)
                n259 = local read "HV 3"() -> (w408:dbl)
                n260 = local write "HV 3"(w399) -> ()
                n261 = Multiply(x=w408, y=w409) -> (x*y=w410:dbl)
                n262 = Multiply(x=w410, y=w401) -> (x*y=w411:dbl)
                n263 = property on="HeatingValueLP 3" class="DigNum (strict)"("Visible"=w396) -> ()  [unwired: 2 in, 2 out]
                n264 = property on="HeatingValueNG 3" class="DigNum (strict)"("Visible"=w397) -> ()  [unwired: 2 in, 2 out]
                n265 = local write "Flow Rate 3"(w411) -> ()
                n266 = local write "Signal 3"(TRUE) -> ()
              }
              frame 2 {
                n267 = local read "Meter Type 6"() -> (w444:string)
                n268 = local read "Meter Type 6"() -> (w441:string)
                n269 = case shown="\"LP\"" w444 {
                  tunnel: [w461 w472] -> w443
                  tunnel: [TRUE FALSE] -> w437
                  tunnel: [FALSE TRUE] -> w438
                  tunnel: [1.0 0.995] -> w442
                  tunnel: [w455 w466] -> w436
                  tunnel: [w454 w465] -> w440
                  frame "LP" {
                    n270 = local read "Meter 6 Size"() -> (w463:dbl)
                    n271 = Divide(x=w463, y=0.5) -> (x/y=w456:dbl)
                    n272 = Multiply(x=0.211888, y=w456) -> (x*y=w461:dbl)
                    n273 = local read "HeatingValueLP 3"() -> (w454:dbl)
                    n274 = Multiply(x=w456, y=2600) -> (x*y=w455:dbl)
                  }
                  frame "NG", Default {
                    n275 = local read "Meter 5 Size"() -> (w474:dbl)
                    n276 = Divide(x=w474, y=1.0) -> (x/y=w467:dbl)
                    n277 = Multiply(x=0.423776, y=w467) -> (x*y=w472:dbl)
                    n278 = local read "HeatingValueNG 3"() -> (w465:dbl)
                    n279 = Multiply(x=w467, y=2200) -> (x*y=w466:dbl)
                  }
                }
                n280 = local read "Reference6"() -> (w447:dbl)
                n281 = local read "Output 6"() -> (w448:dbl)
                n282 = property on="DisplayChart 3" class="WFChart (strict)"("YScale.Minimum"=0.0) -> ()  [unwired: 2 in, 2 out]
                n283 = local write "Gas 3"(w441) -> ()
                n284 = Divide(x=w448, y=w447) -> (x/y=w445:dbl)
                n285 = Compound Arithmetic op=MULTIPLY(w445, 5.0, w443) -> (w439:dbl)
                n286 = local write "CF/HR 3"(w439) -> ()
                n287 = property on="DisplayChart 3" class="WFChart (strict)"("YScale.Maximum"=w436) -> ()  [unwired: 2 in, 2 out]
                n288 = local read "CF/HR 3"() -> (w450:dbl)
                n289 = local read "HV 3"() -> (w449:dbl)
                n290 = local write "HV 3"(w440) -> ()
                n291 = Multiply(x=w449, y=w450) -> (x*y=w451:dbl)
                n292 = Multiply(x=w451, y=w442) -> (x*y=w452:dbl)
                n293 = property on="HeatingValueLP 3" class="DigNum (strict)"("Visible"=w437) -> ()  [unwired: 2 in, 2 out]
                n294 = property on="HeatingValueNG 3" class="DigNum (strict)"("Visible"=w438) -> ()  [unwired: 2 in, 2 out]
                n295 = local write "Flow Rate 3"(w452) -> ()
                n296 = local write "Signal 3"(TRUE) -> ()
              }
            }
          }
          frame #3 {
            n297 = Delete From Array(array=w500, index=599) -> (array with subset deleted=w495:dbl[])  [unwired: 1 in, 1 out]
            n298 = Delete From Array(array=w484, index=399) -> (array with subset deleted=w482:dbl[])  [unwired: 1 in, 1 out]
            n299 = Delete From Array(array=w499, index=1199) -> (array with subset deleted=w496:dbl[])  [unwired: 1 in, 1 out]
            n300 = local read "Flow Rate"() -> (w477:dbl)
            n301 = Insert Into Array(array=w482, index=0, new element=w477) -> (w481:dbl[])
            n302 = Insert Into Array(array=w495, index=0, new element=w477) -> (w494:dbl[])
            n303 = Insert Into Array(array=w496, index=0, new element=w477) -> (w490:dbl[])
            n304 = Add Array Elements(numeric array=w481) -> (sum=w480:dbl)
            n305 = Array Size(array=w481) -> (size(s)=w479:i32)
            n306 = Add Array Elements(numeric array=w490) -> (sum=w489:dbl)
            n307 = Array Size(array=w490) -> (size(s)=w488:i32)
            n308 = Add Array Elements(numeric array=w494) -> (sum=w492:dbl)
            n309 = Array Size(array=w494) -> (size(s)=w493:i32)
            n310 = Divide(x=w480, y=w479) -> (x/y=w478:dbl)
            n311 = Divide(x=w489, y=w488) -> (x/y=w487:dbl)
            n312 = Divide(x=w492, y=w493) -> (x/y=w491:dbl)
            n313 = local write "15 Second Average (BTU/hr)"(w491) -> ()
            n314 = local write "ANSI Placeholder"(w478) -> ()
            n315 = local write "30 Second Average (BTU/hr)"(w487) -> ()
          }
          frame #4 {
            n316 = Delete From Array(array=w517, index=1199) -> (array with subset deleted=w516:dbl[])  [unwired: 1 in, 1 out]
            n317 = Delete From Array(array=w523, index=599) -> (array with subset deleted=w522:dbl[])  [unwired: 1 in, 1 out]
            n318 = Delete From Array(array=w515, index=399) -> (array with subset deleted=w514:dbl[])  [unwired: 1 in, 1 out]
            n319 = local read "Flow Rate 2"() -> (w504:dbl)
            n320 = Insert Into Array(array=w516, index=0, new element=w504) -> (w509:dbl[])
            n321 = Insert Into Array(array=w522, index=0, new element=w504) -> (w510:dbl[])
            n322 = Insert Into Array(array=w514, index=0, new element=w504) -> (w508:dbl[])
            n323 = Add Array Elements(numeric array=w509) -> (sum=w520:dbl)
            n324 = Array Size(array=w509) -> (size(s)=w521:i32)
            n325 = Add Array Elements(numeric array=w510) -> (sum=w524:dbl)
            n326 = Array Size(array=w510) -> (size(s)=w525:i32)
            n327 = Add Array Elements(numeric array=w508) -> (sum=w518:dbl)
            n328 = Array Size(array=w508) -> (size(s)=w519:i32)
            n329 = Divide(x=w520, y=w521) -> (x/y=w503:dbl)
            n330 = Divide(x=w524, y=w525) -> (x/y=w502:dbl)
            n331 = Divide(x=w518, y=w519) -> (x/y=w501:dbl)
            n332 = local write "30 Second Average (BTU/hr) 2"(w503) -> ()
            n333 = local write "15 Second Average (BTU/hr) 2"(w502) -> ()
            n334 = local write "ANSI Placeholder 2"(w501) -> ()
          }
          frame #5 {
            n335 = local read "Flow Rate 3"() -> (w535:dbl)
            n336 = Delete From Array(array=w541, index=1199) -> (array with subset deleted=w540:dbl[])  [unwired: 1 in, 1 out]
            n337 = Delete From Array(array=w538, index=399) -> (array with subset deleted=w537:dbl[])  [unwired: 1 in, 1 out]
            n338 = Delete From Array(array=w544, index=599) -> (array with subset deleted=w543:dbl[])  [unwired: 1 in, 1 out]
            n339 = Insert Into Array(array=w540, index=0, new element=w535) -> (w539:dbl[])
            n340 = Insert Into Array(array=w537, index=0, new element=w535) -> (w536:dbl[])
            n341 = Insert Into Array(array=w543, index=0, new element=w535) -> (w542:dbl[])
            n342 = Add Array Elements(numeric array=w539) -> (sum=w547:dbl)
            n343 = Add Array Elements(numeric array=w536) -> (sum=w545:dbl)
            n344 = Add Array Elements(numeric array=w542) -> (sum=w549:dbl)
            n345 = Array Size(array=w539) -> (size(s)=w548:i32)
            n346 = Array Size(array=w536) -> (size(s)=w546:i32)
            n347 = Array Size(array=w542) -> (size(s)=w550:i32)
            n348 = Divide(x=w547, y=w548) -> (x/y=w533:dbl)
            n349 = Divide(x=w545, y=w546) -> (x/y=w532:dbl)
            n350 = Divide(x=w549, y=w550) -> (x/y=w534:dbl)
            n351 = local write "30 Second Average (BTU/hr) 3"(w533) -> ()
            n352 = local write "15 Second Average (BTU/hr) 3"(w534) -> ()
            n353 = local write "ANSI Placeholder 3"(w532) -> ()
          }
          frame #6 {
            n354 = local read "Start ANSI"() -> (w551:bool)
            n355 = case shown="True" w551 {
              frame False {
              }
              frame True {
                n356 = local read "Start Time ANSI"() -> (w553:dbl)
                n357 = Equal?(x=w553, y=0.0) -> (x = y?=w552:bool)
                n358 = case shown="True" w552 {
                  frame False {
                    n359 = local read "Start Time ANSI"() -> (w559:dbl)
                    n360 = local read "Time"() -> (w556:dbl)
                    n361 = Add(x=w559, y=310) -> (x+y=w557:dbl)
                    n362 = Less Or Equal?(x=w556, y=w557) -> (x <= y?=w555:bool)
                    n363 = case shown="False" w555 {
                      frame False {
                        n364 = local read "ANSI Placeholder"() -> (w561:dbl)
                        n365 = local write "Start Time ANSI"(0.0) -> ()
                        n366 = local write "Start ANSI"(FALSE) -> ()
                        n367 = local write "ANSI Average (BTU/hr)"(w561) -> ()
                      }
                      frame True {
                      }
                    }
                  }
                  frame True {
                    n368 = local read "Time"() -> (w564:dbl)
                    n369 = local write "ANSI Average (BTU/hr)"(0.0) -> ()
                    n370 = local write "Start Time ANSI"(w564) -> ()
                  }
                }
              }
            }
          }
          frame #7 {
            n371 = local read "Start ANSI 2"() -> (w565:bool)
            n372 = case shown="True" w565 {
              frame False {
              }
              frame True {
                n373 = local read "Start Time ANSI 2"() -> (w567:dbl)
                n374 = Equal?(x=w567, y=0.0) -> (x = y?=w566:bool)
                n375 = case shown="False" w566 {
                  frame False {
                    n376 = local read "Start Time ANSI 2"() -> (w573:dbl)
                    n377 = local read "Time"() -> (w570:dbl)
                    n378 = Add(x=w573, y=310) -> (x+y=w571:dbl)
                    n379 = Less Or Equal?(x=w570, y=w571) -> (x <= y?=w569:bool)
                    n380 = case shown="False" w569 {
                      frame False {
                        n381 = local read "ANSI Placeholder 2"() -> (w575:dbl)
                        n382 = local write "Start Time ANSI 2"(0.0) -> ()
                        n383 = local write "Start ANSI 2"(FALSE) -> ()
                        n384 = local write "ANSI Average (BTU/hr) 2"(w575) -> ()
                      }
                      frame True {
                      }
                    }
                  }
                  frame True {
                    n385 = local read "Time"() -> (w578:dbl)
                    n386 = local write "ANSI Average (BTU/hr) 2"(0.0) -> ()
                    n387 = local write "Start Time ANSI 2"(w578) -> ()
                  }
                }
              }
            }
          }
          frame #8 {
            n388 = local read "Start ANSI 3"() -> (w579:bool)
            n389 = case shown="True" w579 {
              frame False {
              }
              frame True {
                n390 = local read "Start Time ANSI 3"() -> (w581:dbl)
                n391 = Equal?(x=w581, y=0.0) -> (x = y?=w580:bool)
                n392 = case shown="False" w580 {
                  frame False {
                    n393 = local read "Start Time ANSI 3"() -> (w587:dbl)
                    n394 = local read "Time"() -> (w584:dbl)
                    n395 = Add(x=w587, y=310) -> (x+y=w585:dbl)
                    n396 = Less Or Equal?(x=w584, y=w585) -> (x <= y?=w583:bool)
                    n397 = case shown="False" w583 {
                      frame False {
                        n398 = local read "ANSI Placeholder 3"() -> (w589:dbl)
                        n399 = local write "Start Time ANSI 3"(0.0) -> ()
                        n400 = local write "Start ANSI 3"(FALSE) -> ()
                        n401 = local write "ANSI Average (BTU/hr) 3"(w589) -> ()
                      }
                      frame True {
                      }
                    }
                  }
                  frame True {
                    n402 = local read "Time"() -> (w592:dbl)
                    n403 = local write "ANSI Average (BTU/hr) 3"(0.0) -> ()
                    n404 = local write "Start Time ANSI 3"(w592) -> ()
                  }
                }
              }
            }
          }
        }
        n405 = local read "Record"() -> (w212:bool)
        n406 = local read "Flow Rate"() -> (w214:dbl)
        n407 = case shown="True" w212 {
          tunnel: w208 -> [w593 w595]
          tunnel: [w593 w594] -> w207
          frame False {
          }
          frame True {
            n408 = Enqueue Element(queue=w595, element="Write to File") -> (queue out=w594:refnum<queue>)  [unwired: 2 in, 2 out]
          }
        }
        n409 = call-poly <vilib>:"DAQmx Read.vi"("task/channels in"=w206) -> ("data"=w205:dbl[])  [unwired: 12 in, 2 out]
        n410 = Bundle("Flow Rate"=w214) -> (→"DisplayChart":cluster{"Flow Rate":dbl})  [unwired: 1 in]
        n411 = Index Array(array=w205, index=8) -> (element=w189:dbl)
        n412 = Index Array(array=w205, index=5) -> (element=w186:dbl)
        n413 = Index Array(array=w205, index=6) -> (element=w187:dbl)
        n414 = Index Array(array=w205, index=7) -> (element=w188:dbl)
        n415 = Index Array(array=w205, index=4) -> (element=w185:dbl)
        n416 = Index Array(array=w205, index=0) -> (element=w181:dbl)
        n417 = Index Array(array=w205, index=1) -> (element=w182:dbl)
        n418 = Index Array(array=w205, index=3) -> (element=w184:dbl)
        n419 = Index Array(array=w205, index=2) -> (element=w183:dbl)
        n420 = local write "Output 3"(w189) -> ()
        n421 = local write "Output 2"(w188) -> ()
        n422 = local write "Output 1"(w187) -> ()
        n423 = local write "Reference1"(w181) -> ()
        n424 = local write "Reference6"(w186) -> ()
        n425 = local write "Reference2"(w182) -> ()
        n426 = local write "Reference4"(w184) -> ()
        n427 = local write "Reference3"(w183) -> ()
        n428 = local write "Reference5"(w185) -> ()
        n429 = local read "Time"() -> (w210:dbl)
        n430 = Add(x=w210, y=0.025) -> (x+y=w209:dbl)
        n431 = Index Array(array=w205, index=9) -> (element=w190:dbl)
        n432 = Index Array(array=w205, index=11) -> (element=w192:dbl)
        n433 = Index Array(array=w205, index=10) -> (element=w191:dbl)
        n434 = local write "Time"(w209) -> ()
        n435 = local read "Flow Rate 2"() -> (w162:dbl)
        n436 = local read "Flow Rate 3"() -> (w161:dbl)
        n437 = local write "Output 6"(w192) -> ()
        n438 = local write "Output 5"(w191) -> ()
        n439 = local write "Output 4"(w190) -> ()
        n440 = Bundle("Flow Rate 2"=w162) -> (→"DisplayChart 2":cluster{"Flow Rate 2":dbl})  [unwired: 1 in]
        n441 = Bundle("Flow Rate 3"=w161) -> (→"DisplayChart 3":cluster{"Flow Rate 3":dbl})  [unwired: 1 in]
      }
    }
  }
  n442 = while {
    shift-right: [w600] -> _
    shift-left: w11 -> [w597]
    shift-right: [w599] -> _
    shift-left: _ -> [w598]
    stop <- FALSE stop-if-true
    n443 = Dequeue Element(queue=w597) -> (element=w601:string)  [unwired: 2 in, 3 out]
    n444 = case shown="\"Write to File\"" w601 {
      tunnel: [w624 w680 w691 w694] -> w600
      tunnel: w597 -> [w624 w680 w691 w694]
      tunnel: [w623 w678 w690 w693] -> w599
      tunnel: w598 -> [_ w679 w690 w693]
      frame "Create File" {
        n445 = Get Date/Time String(date format (0)=1) -> (date string=w629:string, time string=w626:string)  [unwired: 2 in]
        n446 = Search and Replace String(input string=w626, search string=":", replace string="") -> (result string=w635:string)  [unwired: 5 in, 3 out]
        n447 = Search and Replace String(replace all?=TRUE, input string=w629, search string=",", replace string="") -> (result string=w636:string)  [unwired: 4 in, 3 out]
        n448 = Build Array("Time (s)", "Gas Meter", "HV", "CF/HR", "Flow Rate (BTU/hr)", "15 Second Avg Flow Rate (BTU/hr)", "30 Second Avg Flow Rate (BTU/hr)", "ANSI Average (BTU/hr)", "Start ANSI (1=yes, 2=no)", "Gas Meter", "HV", "CF/HR", "Flow Rate (BTU/hr)", "15 Second Avg Flow Rate (BTU/hr)", "30 Second Avg Flow Rate (BTU/hr)", "ANSI Average (BTU/hr)", "Start ANSI (1=yes, 2=no)", "Gas Meter", "HV", "CF/HR", "Flow Rate (BTU/hr)", "15 Second Avg Flow Rate (BTU/hr)", "30 Second Avg Flow Rate (BTU/hr)", "ANSI Average (BTU/hr)", "Start ANSI (1=yes, 2=no)") -> (w646:string[])
        n449 = Concatenate Strings("C:\\Gas Flow Meter\\", w636, " ", w635, ".csv") -> (w632:string)
        n450 = String To Path(string=w632) -> (path=w652:path)
        n451 = Array To Spreadsheet String(delimiter (Tab)=",", array=w646, 3:"%f" ("format string")) -> (spreadsheet string=w647:string)
        n452 = Open/Create/Replace File(file path (use dialog)=w652, operation (0:open)=T1."replace or create", access (0:read/write)=enum16{"read/write", "read-only", "write-only"}."read/write") -> (refnum out=w654:refnum<file>)  [unwired: 3 in, 2 out]
        n453 = local write "Num Record"(1.0) -> ()
        n454 = Refnum to Path(1:w654) -> (0:w653:path)
        n455 = local write "File Path"(w653) -> ()
        n456 = Write to Text File(file (use dialog)=w654, text=w647) -> (refnum out=w623:refnum<file>)  [unwired: 2 in, 2 out]
        n457 = local write "Time"(0.0) -> ()
      }
      frame "Write to File" {
        n458 = local read "30 Second Average (BTU/hr) 2"() -> (w665:dbl)
        n459 = local read "ANSI Average (BTU/hr) 2"() -> (w664:dbl)
        n460 = local read "15 Second Average (BTU/hr) 2"() -> (w666:dbl)
        n461 = local read "15 Second Average (BTU/hr) 3"() -> (w658:dbl)
        n462 = local read "30 Second Average (BTU/hr) 3"() -> (w657:dbl)
        n463 = local read "ANSI Average (BTU/hr) 3"() -> (w656:dbl)
        n464 = local read "Start ANSI 2"() -> (w671:bool)
        n465 = local read "Flow Rate 2"() -> (w667:dbl)
        n466 = local read "Start ANSI 3"() -> (w672:bool)
        n467 = local read "CF/HR 2"() -> (w668:dbl)
        n468 = local read "Flow Rate 3"() -> (w659:dbl)
        n469 = local read "Meter ID 3"() -> (w662:dbl)
        n470 = local read "HV 2"() -> (w669:dbl)
        n471 = local read "Meter ID 2"() -> (w670:dbl)
        n472 = local read "15 Second Average (BTU/hr)"() -> (w676:dbl)
        n473 = local read "CF/HR 3"() -> (w660:dbl)
        n474 = local read "Flow Rate"() -> (w683:dbl)
        n475 = local read "30 Second Average (BTU/hr)"() -> (w677:dbl)
        n476 = local read "Meter ID"() -> (w686:dbl)
        n477 = local read "Start ANSI"() -> (w674:bool)
        n478 = local read "CF/HR"() -> (w684:dbl)
        n479 = local read "HV 3"() -> (w661:dbl)
        n480 = local read "Time"() -> (w687:dbl)
        n481 = local read "HV"() -> (w685:dbl)
        n482 = local read "ANSI Average (BTU/hr)"() -> (w675:dbl)
        n483 = Boolean To (0,1)(Boolean=w672) -> (0, 1=w655:i16)
        n484 = Boolean To (0,1)(Boolean=w671) -> (0, 1=w663:i16)
        n485 = Boolean To (0,1)(Boolean=w674) -> (0, 1=w673:i16)
        n486 = Build Array(w687, w686, w685, w684, w683, w676, w677, w675, w673, w670, w669, w668, w667, w666, w665, w664, w663, w662, w661, w660, w659, w658, w657, w656, w655) -> (w682:dbl[])
        n487 = Array To Spreadsheet String(delimiter (Tab)=",", array=w682, 3:"%.3f" ("format string")) -> (spreadsheet string=w681:string)
        n488 = Write to Text File(file (use dialog)=w679, text=w681) -> (refnum out=w678:refnum<file>)  [unwired: 2 in, 2 out]
      }
      frame "Close File" {
        n489 = Close File(refnum=w690) -> ()  [unwired: 1 in, 2 out]
        n490 = local write "Num Record"(0.0) -> ()
      }
      frame "Initialize", Default {
      }
    }
  }
